vi "LaunchUnitTests.vi"   [LabVIEW 2020]
uses:
  <vilib>/utf/NI_UnitTestFramework.lvlib
  <vilib>/utf/dialogs/utf_testsuite_report_type.ctl
  <vilib>/NI/UTF Junit Report/utf junit report.lvlib
types:
  T1 = typedef "NI_UnitTestFramework.lvlib/utf_testsuite_report_type.ctl" = u16
  T2 = typedef "NI_UnitTestFramework.lvlib/utf_test_result_overall.ctl" = cluster{"utf results out":T3[], "untested VIs":cluster{"VI path":path, "code coverage":T12, "vi hierarchy":string[]}[], "project file path":path, "system information":string}
  T3 = typedef "NI_UnitTestFramework.lvlib/utf_test_result_testfile.ctl" = cluster{"test case":T4[], "test status":T5, "test path":path, "setup VI":path, "teardown VI":path, "code coverage":T12, "start time":timestamp, "end time":timestamp, "test hierarchy":string[], "VI path":path, "VI timestamp":timestamp, "VI rev hist":i32, "requirements ID":string, "array brackets":string, "name separator":string, "errors":T13[], "paragraph header":string, "result comment":string, "vi hierarchy":string[], "subVI coverage info":T12[], "subVI info":T15[], "big array threshold":u32, "VI Index":i32, "Comment":string, "Dynamic Dispatch":bool, "User-defined test VI":path, "user-defined VI code coverage":T12}
  T4 = typedef "NI_UnitTestFramework.lvlib/utf_test_result_testcase.ctl" = cluster{"test result":T5, "run Times":T6[], "test case name":string, "requirements":string, "code coverage":T12, "subVI coverage info":T12[]}
  T5 = typedef "NI_UnitTestFramework.lvlib/utf_test_result.ctl" = enum16{"Passed", "Failed", "Error", "Skipped", "Not Processed"}
  T6 = typedef "NI_UnitTestFramework.lvlib/utf_test_result_troll_new.ctl" = cluster{"result (test)":T5, "Vector Result":T7[]}
  T7 = typedef "NI_UnitTestFramework.lvlib/utf_vector_result.ctl" = cluster{"time elapsed [ms]":u32, "result (test)":T5, "result (parameters)":T8[], "Used Vector Values":cluster{"Vector Name":string, "element":i32}[], "Executed Class Path":path, "Input":T11[]}
  T8 = typedef "NI_UnitTestFramework.lvlib/utf_test_result_failure.ctl" = cluster{"result":T5, "error message":string, "parameter name":string, "parameter value":variant, "parameters":variant[], "comparison":T9, "requirement ID":string, "VI":T10, "Used Vector Name":string}
  T9 = typedef "NI_UnitTestFramework.lvlib/utf_test_comparison_operators.ctl" = enum16{"=", "!=", ">", ">=", "<", "<=", "range", "symmetric tolerance", "asymmetric tolerance", "string contains", "string not contain", "array size", "string length", "array range", "by element", "array range (limit array)", "user-defined", "array contains", "array not contain", "vector length", "= (elm)", "!= (elm)", "= (case insensitive)", "!= (case insensitive)"}
  T10 = typedef "NI_UnitTestFramework.lvlib/utf_vi_tag.ctl" = enum16{"Setup VI", "VI under Test", "Teardown VI"}
  T11 = typedef "NI_UnitTestFramework.lvlib/utf_test_result_input_data.ctl" = cluster{"Name":string, "Input Value":variant[], "VI":T10, "Used Vector Index":i32}
  T12 = typedef "NI_UnitTestFramework.lvlib/utf_code_coverage.ctl" = cluster{"coverage":dbl, "diagram run flag":bool[]}
  T13 = typedef "NI_UnitTestFramework.lvlib/utf_error_data.ctl" = cluster{"error type":T14, "description":string}
  T14 = typedef "NI_UnitTestFramework.lvlib/utf_error_type.ctl" = enum16{"TestFileError", "VIError", "SetupVIError", "TearDownVIError", "OtherError"}
  T15 = typedef "NI_UnitTestFramework.lvlib/utf_subvi_info.ctl" = cluster{"Path":path, "Dependence VI":bool}
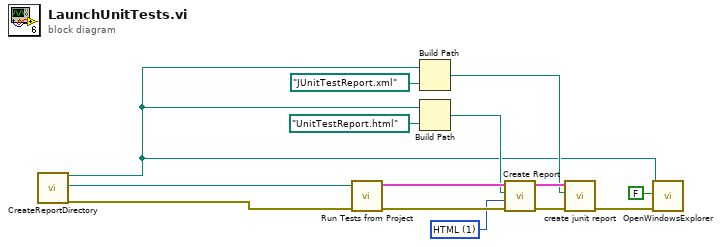
[diagram p0: block diagram]
diagram:
  w12 = T1 1 items=["ASCII (tab-delimited)", "HTML", "ATML (XML-based)"] ("report type (HTML)")
  n1 = call "CreateReportDirectory.vi"() -> ("ReportDirectory"=w1:path, "ProjectFile"=w4:path, "error out"=w3:errorcluster)  [unwired: 17 in]
  n2 = call <vilib>:"Run Tests from Project.vi"("error in (no error)"=w3, "project file path"=w4) -> ("error out"=w13:errorcluster, "test results out"=w14:T2)  [unwired: 8 in]
  n3 = Build Path(base path=w1, name or relative path=path "JUnitTestReport.xml") -> (appended path=w6:path)
  n4 = Build Path(base path=w1, name or relative path=path "UnitTestReport.html") -> (appended path=w8:path)
  n5 = call <vilib>:"Create Report.vi"("error in (no error)"=w13, "report type (HTML)"=w12, "report path"=w8, "test results in"=w14) -> ("error out"=w9:errorcluster, "test results out"=w10:T2)  [unwired: 6 in]
  n6 = call <vilib>:"create junit report.vi"("Error In (No Error)"=w9, "junit report file path"=w6, "test results"=w10) -> ("Error Out"=w2:errorcluster)  [unwired: 8 in]
  n7 = call "OpenWindowsExplorer.vi"("Directory or File"=w1, "Select Directory? (F: Open Directory)"=FALSE, "error in (no error)"=w2) -> ()  [unwired: 16 in, 1 out]
